vi "Tell.vi"(4 "Priority":bool, 10 "Msg":refnum<class "Msg.lvclass">, 11 "Queue Transport in":refnum<class "Queue Transport.lvclass">) -> (0 "Error out":errorcluster)   [LabVIEW 2025, in "jettl.lvlib" / "Transport.lvlib" / "Queue Transport.lvclass"]
uses:
  Queue Transport.lvclass
  Msg/Msg.lvclass
  Queue Transport.lvclass/Queue Transport.ctl
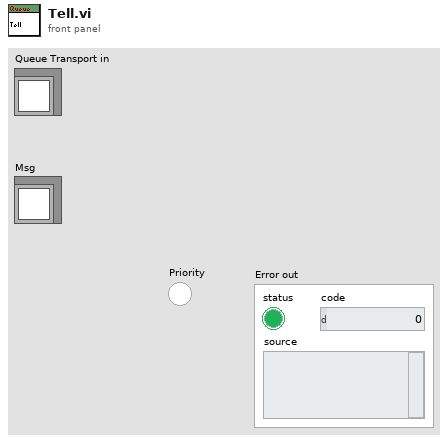
[diagram p1: front panel]
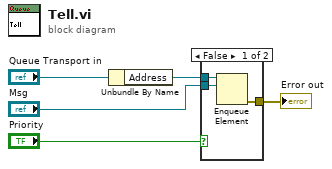
[diagram p0: block diagram]
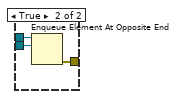
[diagram p2: hidden frame]
diagram:
  n1 = Unbundle By Name("Queue Transport in") -> ("Address"=w4:refnum<queue>)
  n2 = case shown="False" "Priority" {
    tunnel: w4 -> [w8 w11]
    tunnel: [w7 w9] -> w3
    tunnel: "Msg" -> [w6 w10]
    frame False {
      n3 = Enqueue Element(queue=w8, element=w6) -> (error out=w7:errorcluster)  [unwired: 2 in, 2 out]
    }
    frame True {
      n4 = Enqueue Element At Opposite End(queue=w11, element=w10) -> (error out=w9:errorcluster)  [unwired: 2 in, 2 out]
    }
  }
  "Error out" <- w3
